vi "Protocol.Send Reset Previously Active DTC to Main.vi"(8 "error in (no error)":errorcluster, 10 "Address":u8, 11 "Simulated Addresses LUT":variant) -> (0 "error out":errorcluster, 2 "found":bool)   [LabVIEW 2019, in "J1939 Addon Engine.lvlib"]
uses:
  J1939 Addon Engine.lvlib
  Types/Engine.Node DTC Settings.ctl
  Addon Shared/Types/Monitor Settings.ctl
  Types/Engine.DTC Settings.ctl
  Addon Shared/Types/Compiled Simulated Settings.ctl
  <vilib>/NI VeriStand/Custom Device API/Block Data Reference.ctl
  <vilib>/NI VeriStand/Custom Device API/Data Reference.ctl
  Types/Engine.DTC FIFOs.ctl
  <vilib>/NI VeriStand/Custom Device API/Custom Device API.lvlib
  Addon Shared/J1939 Addon Shared.lvlib
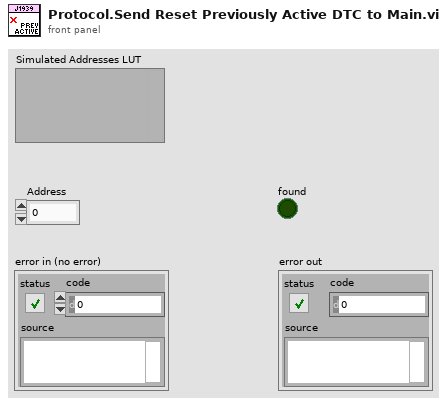
[diagram p1: front panel]
types:
  T1 = typedef "J1939 Addon Engine.lvlib/Engine.Node DTC Settings.ctl" = cluster{"Network":T2, "Sim DTC Refs":T3}
  T2 = typedef "J1939 Addon Shared.lvlib/Monitor Settings.ctl" = cluster{"Address":u8, "Name":u64, "Include DA":bool}
  T3 = typedef "J1939 Addon Engine.lvlib/Engine.DTC Settings.ctl" = cluster{"Data":T4, "FIFOs":T7}
  T4 = typedef "J1939 Addon Shared.lvlib/Compiled Simulated Settings.ctl" = cluster{"DM1.Ref":T5[], "DM1.Value":dbl[], "DM1.Enable.Ref":T5[], "DM1.Enable.Value":dbl[], "DM2.Ref":T5[], "DM2.Value":dbl[], "DM2.Enable.Ref":T5[], "DM2.Enable.Value":dbl[]}
  T5 = typedef "Custom Device API.lvlib/Block Data Reference.ctl" = cluster{"Data Reference":T6, "Offset":u64, "Length":u64}
  T6 = typedef "Custom Device API.lvlib/Data Reference.ctl" = i32
  T7 = typedef "J1939 Addon Engine.lvlib/Engine.DTC FIFOs.ctl" = cluster{"DM1.Data":refnum<k33>, "DM1.Enable":refnum<k33>, "DM2.Data":refnum<k33>, "DM2.Enable":refnum<k33>, "DM1.Reset":refnum<k33>, "DM2.Reset":refnum<k33>}
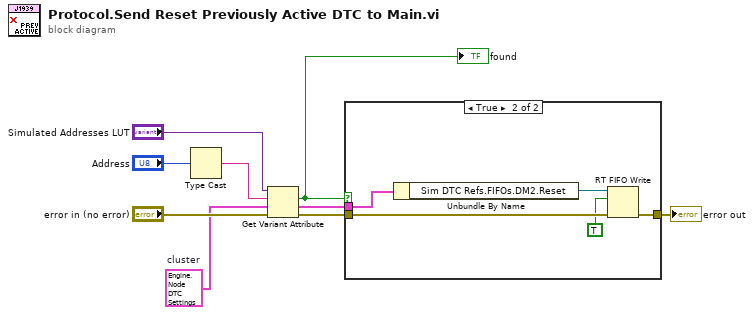
[diagram p0: block diagram]
diagram:
  w1 = T1 {"Network"={"Address"=0, "Name"=0, "Include DA"=FALSE}, "Sim DTC Refs"={"Data"={"DM1.Ref"=[], "DM1.Value"=[], "DM1.Enable.Ref"=[], "DM1.Enable.Value"=[], "DM2.Ref"=[], "DM2.Value"=[], "DM2.Enable.Ref"=[], "DM2.Enable.Value"=[]}, "FIFOs"={"DM1.Data"=refnum, "DM1.Enable"=refnum, "DM2.Data"=refnum, "DM2.Enable"=refnum, "DM1.Reset"=refnum, "DM2.Reset"=refnum}}}  # cluster
  n1 = Type Cast(x="Address") -> (*(type *) &x=w8:string)  [unwired: 1 in]
  n2 = Get Variant Attribute(Variant="Simulated Addresses LUT", name=w8, default value (empty Variant)=w1, error in="error in (no error)") -> (found=w5:bool, value=w3:T1, error out=w4:errorcluster)  [unwired: 1 out]
  "found" <- w5
  n3 = case shown="True" w5 {
    tunnel: w4 -> [w10 w13]
    tunnel: w3 -> [_ w15]
    tunnel: [w10 w11] -> w2
    frame False {
    }
    frame True {
      n4 = Unbundle By Name(w15) -> ("Sim DTC Refs.FIFOs.DM2.Reset"=w14:refnum<k33>)
      n5 = RT FIFO Write(0:w14, 1:TRUE ("element"), 3:w13) -> (11:w11:errorcluster)  [unwired: 2 in, 3 out]
    }
  }
  "error out" <- w2
